vi "Untitled 2.vi"(8 "error in (no error)":errorcluster, 11 "ACQ Contador in":refnum<class "ACQ Contador.lvclass">) -> (0 "error out":errorcluster, 3 "ACQ Contador out":refnum<class "ACQ Contador.lvclass">)   [LabVIEW 2020]
uses:
  ACQ Contador.lvclass
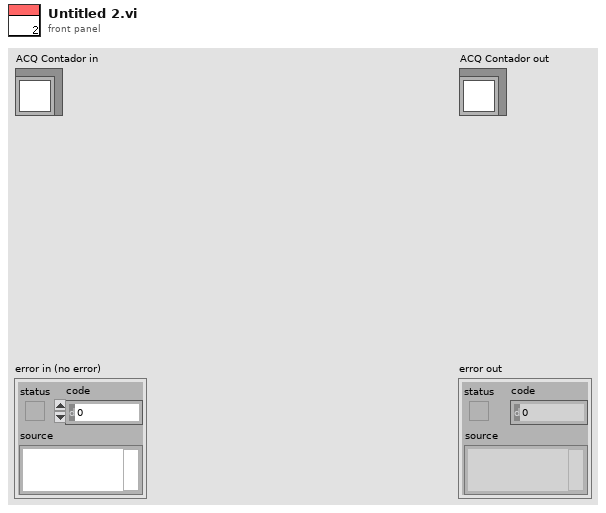
[diagram p1: front panel]
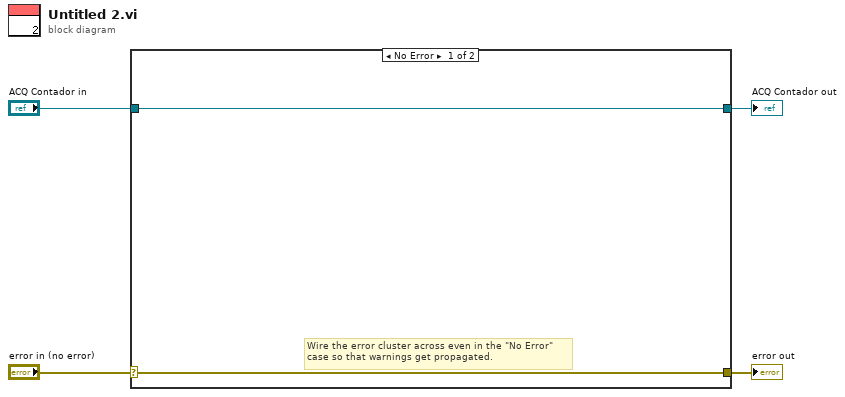
[diagram p0: block diagram]
diagram:
  n1 = case shown="No Error" "error in (no error)" {
    selector: "error in (no error)" -> [w5 w8]
    tunnel: [w5 w8] -> w3
    tunnel: [w6 w7] -> w1
    tunnel: "ACQ Contador in" -> [w6 w7]
    frame No Error {
      # "Wire the error cluster across even in the \"No Error\"\ncase so that warnings get propagated."
    }
    frame Error {
    }
  }
  "error out" <- w3
  "ACQ Contador out" <- w1
